vi "Write Blink.vi"(8 "error in (no error)":errorcluster, 9 "Blink On":bool, 11 "PCF8574 I2C LCD I in":refnum<class "PCF8574 I2C LCD.lvclass">) -> (0 "error out":errorcluster, 3 "PCF8574 I2C LCD I out":refnum<class "PCF8574 I2C LCD.lvclass">)   [LabVIEW 2020, in "CTI-Peripheral.lvlib" / "PCF8574 I2C LCD.lvclass"]
uses:
  PCF8574 I2C LCD.lvclass
  PCF8574 I2C LCD.lvclass/PCF8574 I2C LCD.ctl
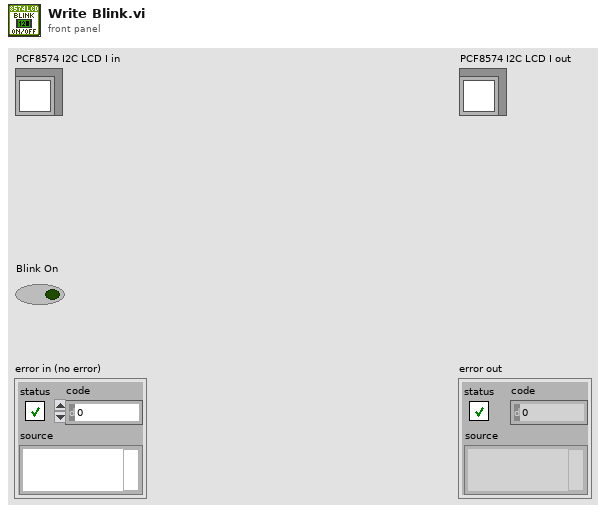
[diagram p1: front panel]
types:
  T1 = typedef "CTI-Peripheral.lvlib/HD44780 LCD.lvlib/Display Control.ctl" = cluster{"Blink On":bool, "Cursor On":bool, "Display On":bool}
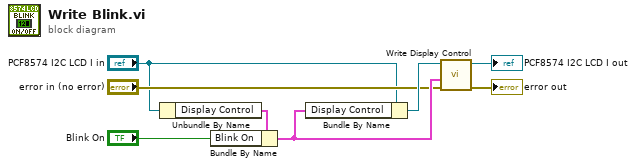
[diagram p0: block diagram]
diagram:
  n1 = Unbundle By Name("PCF8574 I2C LCD I in") -> ("Display Control"=w8:T1)
  n2 = Bundle By Name(cluster=w8, "Blink On"="Blink On") -> (w6:T1)
  n3 = Bundle By Name(cluster="PCF8574 I2C LCD I in", "Display Control"=w6) -> (w7:refnum<class "PCF8574 I2C LCD.lvclass">)
  n4 = call "Write Display Control.vi"("error in (no error)"="error in (no error)", "Display Control"=w6, "PCF8574 I2C LCD in"=w7) -> ("error out"=→"error out":errorcluster, "PCF8574 I2C LCD out"=→"PCF8574 I2C LCD I out":refnum<class "PCF8574 I2C LCD.lvclass">)  [unwired: 7 in]
